vi "NormalBeam.vi"() -> ()   [LabVIEW 2017]
uses:
  <vilib>/Math Plots/2D Math Plots/XY Plot Matrix/XY Plot Matrix XCtrl/XY Plot Matrix.xctl
  <vilib>/ULx/Create Channel.llb/ULx Create Channel (AI-Voltage-Basic).vi
  <vilib>/ULx/Read.llb/ULx Read (Analog Wfm 1Chan NSamp).vi
  <vilib>/Analysis/Matrix/Numeric/Conversions/Array To Matrix - RA.vi
  <vilib>/ULx/Timing.llb/ULx Timing (Sample Clock).vi
  <vilib>/Math Plots/2D Math Plots/XY Plot Matrix/XY Plot Matrix Datatype/XY Plot Matrix Datatype.lvclass
  <vilib>/Analysis/Matrix/NI_Matrix.lvlib
panel:
  out "Weight Scale":dbl[](array[numeric])
  out "XY Plot Matrix":refnum<class "XY Plot Matrix Datatype.lvclass">[](xcontrol)
  out "Number of Sample":dbl format="%.0g"
  out "Voltage":dbl
  out "Array":dbl[](array[numeric])
  in  "Build Array!":bool
  in  "Number of Calibrations":i8
  in  "Maximum Weight":dbl
  in  "Minimum Weight":dbl
  in  "Sample":bool
  out "Waveform Chart":waveform(dbl)(graph)
  out "Waveform Graph":waveform(dbl)(graph)
  in  "rate":dbl=1000.0
  in  "samples per channel":i32=1000
  in  "sample mode":i32(ring) items=["FiniteSamples", "ContinuousSamples"]
  in  "minimum value":dbl=-5.0
  in  "maximum value":dbl=5.0
  in  "physical channels":refnum<k21>
  # "Data size calculator"
  # "What is the range of your calibration?"
  # "How many Calibrations do you want to make?(Times two)"
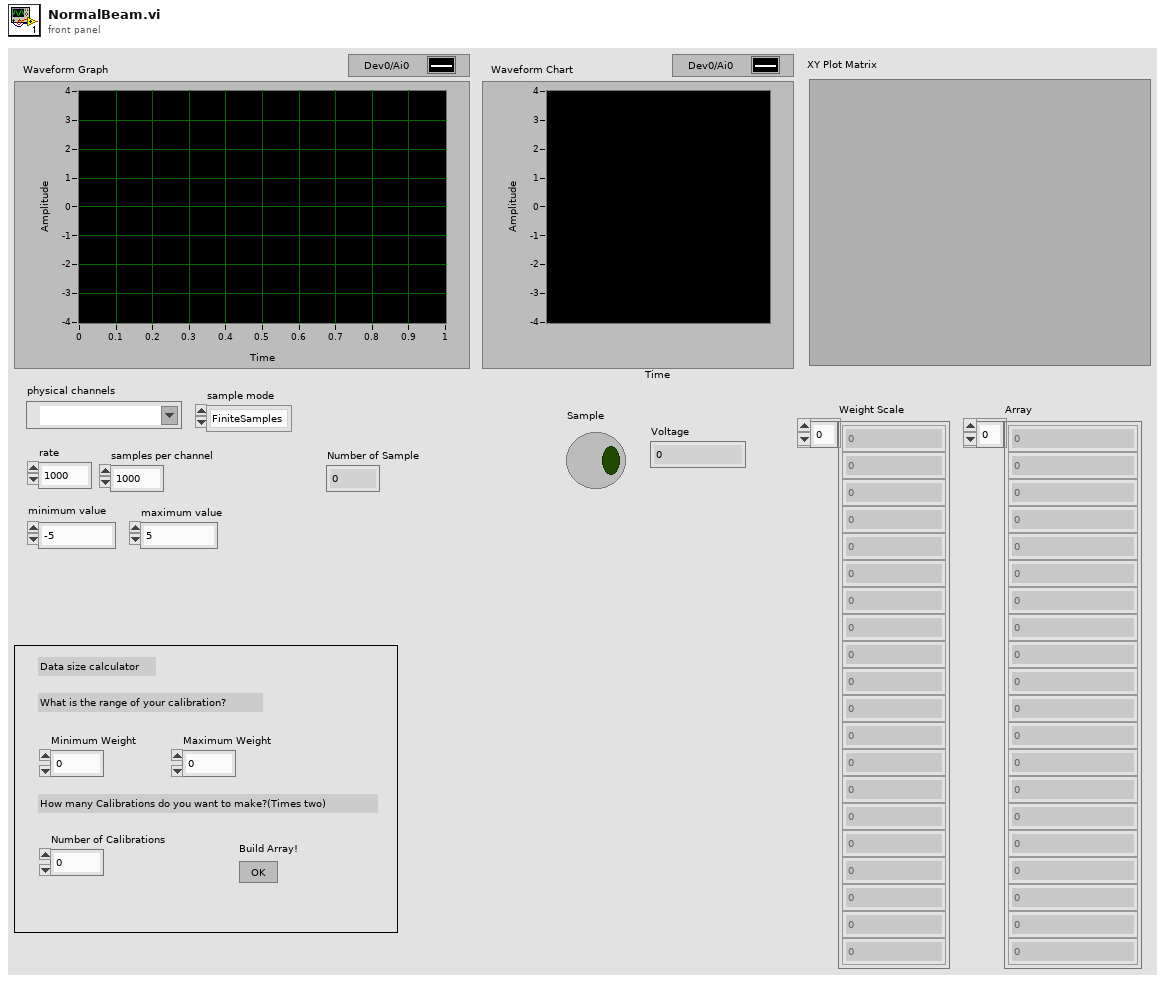
[diagram p1: front panel]
types:
  T1 = typedef "NI_Matrix.lvlib/RealMatrix.ctl" = dbl[][]
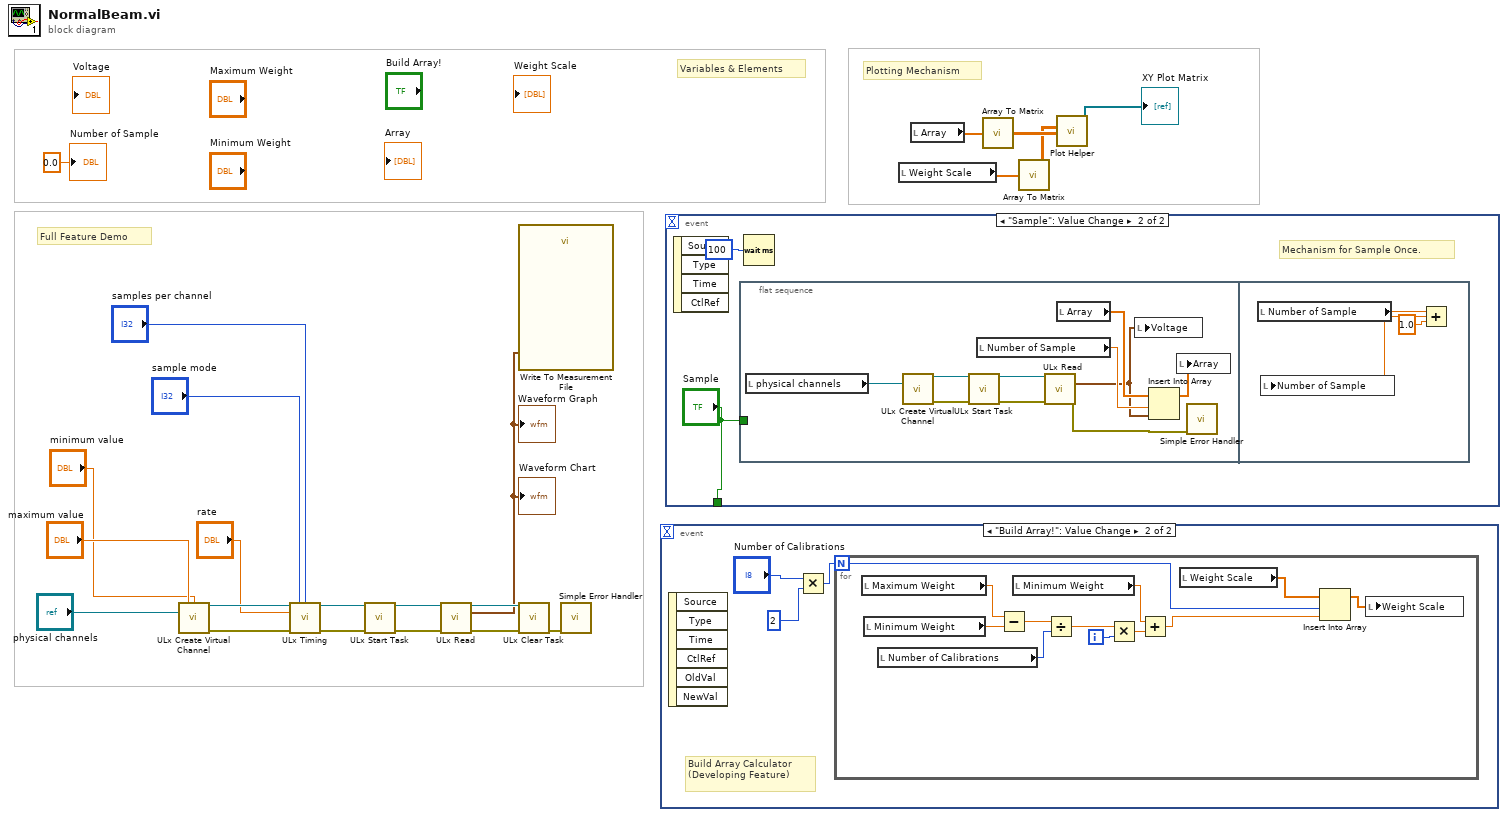
[diagram p0: block diagram]
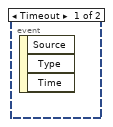
[diagram p2: hidden frame]
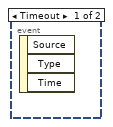
[diagram p3: hidden frame]
diagram:
  # "Full Feature Demo"
  # "Plotting Mechanism"
  # "Variables & Elements"
  n1 = call-poly <vilib>:"ULx Create Virtual Channel.vi"("maximum value"="maximum value", "minimum value"="minimum value", "physical channels"="physical channels") -> ("task out"=w17:refnum<k24>, "error out"=w16:errorcluster)  [unwired: 11 in]
  n2 = call-poly <vilib>:"ULx Timing.vi"("task in"=w17, "sample mode"="sample mode", "samples per channel"="samples per channel", "rate"="rate", "error in"=w16) -> ("task out"=w14:refnum<k24>, "error out"=w13:errorcluster)  [unwired: 9 in]
  n3 = call <vilib>:"ULx Start Task.vi"("task in"=w14, "error in"=w13) -> ("task out"=w12:refnum<k24>, "error out"=w11:errorcluster)  [unwired: 12 in]
  n4 = call-poly <vilib>:"ULx Read.vi"("task in"=w12, "error in"=w11) -> ("task out"=w10:refnum<k24>, "data"=w7:waveform(dbl), "error out"=w9:errorcluster)  [unwired: 11 in]
  "Waveform Graph" <- w7
  "Waveform Chart" <- w7
  n5 = call "Write To Measurement File"("Signals"=w7) -> ()  [unwired: 16 in, 3 out]
  n6 = call <vilib>:"ULx Clear Task.vi"("task in"=w10, "error in"=w9) -> ("error out"=w8:errorcluster)  [unwired: 13 in]
  n7 = call <vilib>:"Simple Error Handler.vi"("error in (no error)"=w8) -> ()  [unwired: 4 in, 5 out]
  n8 = event shown="[1] \"Build Array!\": Value Change" {
    selector: _ -> [_ _]
    dyn-events: _ -> [_ _]
    timeout: _ -> [_ _]
    event Timeout {
      n9 = event-data() -> ()  [unwired: 1 in, 3 out]
    }
    event "Build Array!": Value Change {
      # "Build Array Calculator\n(Developing Feature)"
      n10 = event-data() -> ()  [unwired: 1 in, 6 out]
      n11 = Multiply(x="Number of Calibrations", y=2) -> (x*y=w23:i32)
      n12 = for {
        N: w23 -> [w29]
        i -> [w31]
        n13 = local read "Maximum Weight"() -> (w36:dbl)
        n14 = local read "Minimum Weight"() -> (w35:dbl)
        n15 = local read "Number of Calibrations"() -> (w33:i8)
        n16 = Subtract(x=w36, y=w35) -> (x-y=w34:dbl)
        n17 = local read "Minimum Weight"() -> (w37:dbl)
        n18 = Divide(x=w34, y=w33) -> (x/y=w32:dbl)
        n19 = Multiply(x=w32, y=w31) -> (x*y=w30:dbl)
        n20 = Add(x=w37, y=w30) -> (x+y=w27:dbl)
        n21 = local read "Weight Scale"() -> (w28:dbl[])
        n22 = Insert Into Array(array=w28, index=w29, new element=w27) -> (w26:dbl[])
        n23 = local write "Weight Scale"(w26) -> ()
      }
    }
  }
  n24 = event shown="[1] \"Sample\": Value Change" {
    selector: _ -> [_ _]
    dyn-events: _ -> [_ _]
    timeout: _ -> [_ _]
    tunnel: [_ "Sample"] -> _
    event Timeout {
      n25 = event-data() -> ()  [unwired: 1 in, 3 out]
    }
    event "Sample": Value Change {
      # "Mechanism for Sample Once."
      n26 = event-data() -> ()  [unwired: 1 in, 4 out]
      n27 = flat-sequence {
        tunnel: "Sample" -> [_]
        frame #0 {
          n28 = local read "physical channels"() -> (w46:refnum<k21>)
          n29 = call-poly <vilib>:"ULx Create Virtual Channel.vi"("physical channels"=w46) -> ("task out"=w45:refnum<k24>, "error out"=w42:errorcluster)  [unwired: 13 in]
          n30 = call <vilib>:"ULx Start Task.vi"("task in"=w45, "error in"=w42) -> ("task out"=w44:refnum<k24>, "error out"=w43:errorcluster)  [unwired: 12 in]
          n31 = local read "Number of Sample"() -> (w48:dbl)
          n32 = call-poly <vilib>:"ULx Read.vi"("task in"=w44, "error in"=w43) -> ("data"=w41:waveform(dbl), "error out"=w40:errorcluster)  [unwired: 11 in, 1 out]
          n33 = local read "Array"() -> (w47:dbl[])
          n34 = local write "Voltage"(w41) -> ()
          n35 = Insert Into Array(array=w47, index=w48, new element=w41) -> (w49:dbl[])
          n36 = local write "Array"(w49) -> ()
          n37 = call <vilib>:"Simple Error Handler.vi"("error in (no error)"=w40) -> ()  [unwired: 4 in, 5 out]
        }
        frame #1 {
          n38 = local read "Number of Sample"() -> (w52:dbl)
          n39 = Add(x=w52, y=1.0) -> (x+y=w51:dbl)
          n40 = local write "Number of Sample"(w51) -> ()
        }
      }
      n41 = Wait (ms)(milliseconds to wait=u32 100) -> ()  [unwired: 1 out]
    }
  }
  n42 = local read "Weight Scale"() -> (w3:dbl[])
  n43 = local read "Array"() -> (w4:dbl[])
  n44 = call-poly <vilib>:"Array To Matrix.vi"("Real 1D Array"=w4) -> ("Real Matrix (Column Vector)"=w2:T1)
  n45 = call-poly <vilib>:"Array To Matrix.vi"("Real 1D Array"=w3) -> ("Real Matrix (Column Vector)"=w1:T1)
  n46 = call <vilib>:"Plot Helper.vi"("y matrix"=w2, "x matrix"=w1) -> ("2D Plotmatrix Class Obj Array out"=→"XY Plot Matrix":refnum<class "XY Plot Matrix Datatype.lvclass">[])  [unwired: 2 in, 7 out]
  "Number of Sample" <- 0.0 ("Number of Sample")
